vi "Func-엑셀 데이터를 그래프로 출력.vi"() -> ()   [LabVIEW 2015] (continued)
645.21\n645.23\n645.24\n645.26\n645.28\n645.29\n645.31\n645.33\n645.34\n645.36\n645.38\n645.39\n645.41\n645.43\n645.44\n645.46\n645.48\n645.49\n645.51\n645.53\n645.54\n645.56\n645.58\n645.59\n645.61\n645.63\n645.64\n645.66\n645.68\n645.69\n645.71\n645.73\n645.74\n645.76\n645.78\n645.79\n645.81\n645.83\n645.84\n645.86\n645.88\n645.89\n645.91\n645.93\n645.94\n645.96\n645.98\n645.99\n646.01\n646.03\n646.04\n646.06\n646.08\n646.09\n646.11\n646.13\n646.14\n646.16\n646.18\n646.19\n646.21\n646.23\n646.24\n646.26\n646.28\n646.29\n646.31\n646.33\n646.34\n646.36\n646.38\n646.39\n646.41\n646.43\n646.44\n646.46\n646.48\n646.49\n646.51\n646.53\n646.54\n646.56\n646.58\n646.59\n646.61\n646.63\n646.64\n646.66\n646.68\n646.69\n646.71\n646.73\n646.74\n646.76\n646.78\n646.8\n646.81\n646.83\n646.84\n646.86\n646.88\n646.89\n646.91\n646.93\n646.94\n646.96\n646.98\n646.99\n647.01\n647.03\n647.04\n647.06\n647.08\n647.09\n647.11\n647.13\n647.15\n647.16\n647.18\n647.19\n647.21\n647.23\n647.25\n647.26\n647.28\n647.29\n647.31\n647.33\n647.34\n647.36\n647.38\n647.4\n647.41\n647.43\n647.44\n647.46\n647.48\n647.49\n647.51\n647.53\n647.54\n647.56\n647.58\n647.59\n647.61\n647.63\n647.64\n647.66\n647.68\n647.69\n647.71\n647.73\n647.74\n647.76\n647.78\n647.79\n647.81\n647.83\n647.84\n647.86\n647.88\n647.89\n647.91\n647.93\n647.94\n647.96\n647.98\n647.99\n648.01\n648.03\n648.04\n648.06\n648.08\n648.09\n648.11\n648.13\n648.14\n648.16\n648.18\n648.19\n648.21\n648.23\n648.24\n648.26\n648.28\n648.29\n648.31\n648.33\n648.35\n648.36\n648.38\n648.39\n648.41\n648.43\n648.44\n648.46\n648.48\n648.49\n648.51\n648.53\n648.54\n648.56\n648.58\n648.59\n648.61\n648.63\n648.64\n648.66\n648.68\n648.69\n648.71\n648.73\n648.75\n648.76\n648.78\n648.79\n648.81\n648.83\n648.84\n648.86\n648.88\n648.89\n648.91\n648.93\n648.94\n648.96\n648.98\n648.99\n649.01\n649.03\n649.04\n649.06\n649.08\n649.09\n649.11\n649.13\n649.14\n649.16\n649.18\n649.19\n649.21\n649.23\n649.24\n649.26\n649.28\n649.29\n649.31\n649.33\n649.34\n649.36\n649.38\n649.39\n649.41\n649.43\n649.44\n649.46\n649.48\n649.49\n649.51\n649.53\n649.55\n649.56\n649.58\n649.59\n649.61\n649.63\n649.64\n649.66\n649.68\n649.69\n649.71\n649.73\n649.74\n649.76\n649.78\n649.79\n649.81\n649.83\n649.84\n649.86\n649.88\n649.9\n649.91\n649.93\n649.94\n649.96\n649.98\n649.99\n650.01\n650.03\n650.04\n650.06\n650.08\n650.09\n650.11\n650.13\n650.15\n650.16\n650.18\n650.19\n650.21\n650.23\n650.25\n650.26\n650.28\n650.29\n650.31\n650.33\n650.35\n650.36\n650.38\n650.39\n650.41\n650.43\n650.44\n650.46\n650.48\n650.5\n650.51\n650.53\n650.54\n650.56\n650.58\n650.6\n650.61\n650.63\n650.64\n650.66\n650.68\n650.69\n650.71\n650.73\n650.74\n650.76\n650.78\n650.79\n650.81\n650.83\n650.85\n650.86\n650.88\n650.89\n650.91\n650.93\n650.94\n650.96\n650.98\n650.99\n651.01\n651.03\n651.05\n651.06\n651.08\n651.09\n651.11\n651.13\n651.14\n651.16\n651.18\n651.19\n651.21\n651.23\n651.24\n651.26\n651.28\n651.29\n651.31\n651.33\n651.34\n651.36\n651.38\n651.39\n651.41\n651.43\n651.44\n651.46\n651.48\n651.49\n651.51\n651.53\n651.54\n651.56\n651.58\n651.59\n651.61\n651.63\n651.64\n651.66\n651.68\n651.69\n651.71\n651.73\n651.74\n651.76\n651.78\n651.79\n651.81\n651.83\n651.84\n651.86\n651.88\n651.89\n651.91\n651.93\n651.94\n651.96\n651.98\n651.99\n652.01\n652.03\n652.04\n652.06\n652.08\n652.09\n652.11\n652.13\n652.14\n652.16\n652.18\n652.19\n652.21\n652.23\n652.24\n652.26\n652.28\n652.29\n652.31\n652.33\n652.34\n652.36\n652.38\n652.39\n652.41\n652.43\n652.44\n652.46\n652.48\n652.49\n652.51\n652.53\n652.54\n652.56\n652.58\n652.59\n652.61\n652.63\n652.64\n652.66\n652.68\n652.69\n652.71\n652.73\n652.74\n652.76\n652.78\n652.79\n652.81\n652.83\n652.84\n652.86\n652.88\n652.89\n652.91\n652.93\n652.94\n652.96\n652.98\n653\n653.01\n653.03\n653.04\n653.06\n653.08\n653.09\n653.11\n653.13\n653.14\n653.16\n653.18\n653.19\n653.21\n653.23\n653.24\n653.26\n653.28\n653.29\n653.31\n653.33\n653.35\n653.36\n653.38\n653.39\n653.41\n653.43\n653.44\n653.46\n653.48\n653.49\n653.51\n653.53\n653.54\n653.56\n653.58\n653.6\n653.61\n653.63\n653.64\n653.66\n653.68\n653.7\n653.71\n653.73\n653.74\n653.76\n653.78\n653.79\n653.81\n653.83\n653.84\n653.86\n653.88\n653.89\n653.91\n653.93\n653.94\n653.96\n653.98\n653.99\n654.01\n654.03\n654.04\n654.06\n654.08\n654.09\n654.11\n654.13\n654.15\n654.16\n654.18\n654.19\n654.21\n654.23\n654.24\n654.26\n654.28\n654.3\n654.31\n654.33\n654.34\n654.36\n654.38\n654.39\n654.41\n654.43\n654.44\n654.46\n654.48\n654.49\n654.51\n654.53\n654.54\n654.56\n654.58\n654.59\n654.61\n654.63\n654.64\n654.66\n654.68\n654.69\n654.71\n654.73\n654.74\n654.76\n654.78\n654.79\n654.81\n654.83\n654.84\n654.86\n654.88\n654.89\n654.91\n654.93\n654.94\n654.96\n654.98\n654.99\n655.01\n655.03\n655.04\n655.06\n655.08\n655.09\n655.11\n655.13\n655.14\n655.16\n655.18\n655.19\n655.21\n655.23\n655.24\n655.26\n655.28\n655.29\n655.31\n655.33\n655.34\n655.36\n655.38\n655.39\n655.41\n655.43\n655.44\n655.46\n655.48\n655.49\n655.51\n655.53\n655.54\n655.56\n655.58\n655.59\n655.61\n655.63\n655.65\n655.66\n655.68\n655.69\n655.71\n655.73\n655.74\n655.76\n655.78\n655.79\n655.81\n655.83\n655.84\n655.86\n655.88\n655.89\n655.91\n655.93\n655.94\n655.96\n655.98\n655.99\n656.01\n656.03\n656.04\n656.06\n656.08\n656.1\n656.11\n656.13\n656.14\n656.16\n656.18\n656.19\n656.21\n656.23\n656.25\n656.26\n656.28\n656.29\n656.31\n656.33\n656.35\n656.36\n656.38\n656.39\n656.41\n656.43\n656.45\n656.46\n656.48\n656.49\n656.51\n656.53\n656.54\n656.56\n656.58\n656.59\n656.61\n656.63\n656.64\n656.66\n656.68\n656.7\n656.71\n656.73\n656.74\n656.76\n656.78\n656.8\n656.81\n656.83\n656.84\n656.86\n656.88\n656.89\n656.91\n656.93\n656.94\n656.96\n656.98\n656.99\n657.01\n657.03\n657.05\n657.06\n657.08\n657.09\n657.11\n657.13\n657.14\n657.16\n657.18\n657.19\n657.21\n657.23\n657.24\n657.26\n657.28\n657.29\n657.31\n657.33\n657.34\n657.36\n657.38\n657.39\n657.41\n657.43\n657.44\n657.46\n657.48\n657.49\n657.51\n657.53\n657.54\n657.56\n657.58\n657.6\n657.61\n657.63\n657.64\n657.66\n657.68\n657.69\n657.71\n657.73\n657.74\n657.76\n657.78\n657.79\n657.81\n657.83\n657.84\n657.86\n657.88\n657.89\n657.91\n657.93\n657.94\n657.96\n657.98\n657.99\n658.01\n658.03\n658.04\n658.06\n658.08\n658.09\n658.11\n658.13\n658.14\n658.16\n658.18\n658.19\n658.21\n658.23\n658.24\n658.26\n658.28\n658.29\n658.31\n658.33\n658.34\n658.36\n658.38\n658.39\n658.41\n658.43\n658.44\n658.46\n658.48\n658.49\n658.51\n658.53\n658.54\n658.56\n658.58\n658.59\n658.61\n658.63\n658.64\n658.66\n658.68\n658.69\n658.71\n658.73\n658.74\n658.76\n658.78\n658.79\n658.81\n658.83\n658.84\n658.86\n658.88\n658.89\n658.91\n658.93\n658.94\n658.96\n658.98\n658.99\n659.01\n659.03\n659.04\n659.06\n659.08\n659.09\n659.11\n659.13\n659.14\n659.16\n659.18\n659.2\n659.21\n659.23\n659.24\n659.26\n659.28\n659.29\n659.31\n659.33\n659.34\n659.36\n659.38\n659.39\n659.41\n659.43\n659.45\n659.46\n659.48\n659.49\n659.51\n659.53\n659.54\n659.56\n659.58\n659.59\n659.61\n659.63\n659.64\n659.66\n659.68\n659.69\n659.71\n659.73\n659.74\n659.76\n659.78\n659.8\n659.81\n659.83\n659.84\n659.86\n659.88\n659.9\n659.91\n659.93\n659.94\n659.96\n659.98\n659.99\n660.01\n660.03\n660.04\n660.06\n660.08\n660.09\n660.11\n660.13\n660.14\n660.16\n660.18\n660.19\n660.21\n660.23\n660.24\n660.26\n660.28\n660.29\n660.31\n660.33\n660.34\n660.36\n660.38\n660.39\n660.41\n660.43\n660.44\n660.46\n660.48\n660.5\n660.51\n660.53\n660.54\n660.56\n660.58\n660.59\n660.61\n660.63\n660.65\n660.66\n660.68\n660.69\n660.71\n660.73\n660.74\n660.76\n660.78\n660.79\n660.81\n660.83\n660.84\n660.86\n660.88\n660.89\n660.91\n660.93\n660.94\n660.96\n660.98\n660.99\n661.01\n661.03\n661.04\n661.06\n661.08\n661.09\n661.11\n661.13\n661.14\n661.16\n661.18\n661.19\n661.21\n661.23\n661.24\n661.26\n661.28\n661.29\n661.31\n661.33\n661.34\n661.36\n661.38\n661.39\n661.41\n661.43\n661.44\n661.46\n661.48\n661.49\n661.51\n661.53\n661.54\n661.56\n661.58\n661.59\n661.61\n661.63\n661.64\n661.66\n661.68\n661.69\n661.71\n661.73\n661.75\n661.76\n661.78\n661.79\n661.81\n661.83\n661.84\n661.86\n661.88\n661.89\n661.91\n661.93\n661.94\n661.96\n661.98\n661.99\n662.01\n662.03\n662.04\n662.06\n662.08\n662.09\n662.11\n662.13\n662.14\n662.16\n662.18\n662.2\n662.21\n662.23\n662.24\n662.26\n662.28\n662.29\n662.31\n662.33\n662.35\n662.36\n662.38\n662.39\n662.41\n662.43\n662.45\n662.46\n662.48\n662.49\n662.51\n662.53\n662.55\n662.56\n662.58\n662.59\n662.61\n662.63\n662.64\n662.66\n662.68\n662.69\n662.71\n662.73\n662.74\n662.76\n662.78\n662.8\n662.81\n662.83\n662.84\n662.86\n662.88\n662.9\n662.91\n662.93\n662.95\n662.96\n662.98\n662.99\n663.01\n663.03\n663.04\n663.06\n663.08\n663.09\n663.11\n663.13\n663.15\n663.16\n663.18\n663.19\n663.21\n663.23\n663.24\n663.26\n663.28\n663.29\n663.31\n663.33\n663.34\n663.36\n663.38\n663.4\n663.41\n663.43\n663.44\n663.46\n663.48\n663.49\n663.51\n663.53\n663.54\n663.56\n663.58\n663.59\n663.61\n663.63\n663.64\n663.66\n663.68\n663.7\n663.71\n663.73\n663.74\n663.76\n663.78\n663.79\n663.81\n663.83\n663.84\n663.86\n663.88\n663.89\n663.91\n663.93\n663.94\n663.96\n663.98\n664\n664.01\n664.03\n664.04\n664.06\n664.08\n664.09\n664.11\n664.13\n664.14\n664.16\n664.18\n664.19\n664.21\n664.23\n664.24\n664.26\n664.28\n664.29\n664.31\n664.33\n664.34\n664.36\n664.38\n664.39\n664.41\n664.43\n664.44\n664.46\n664.48\n664.49\n664.51\n664.53\n664.54\n664.56\n664.58\n664.59\n664.61\n664.63\n664.64\n664.66\n664.68\n664.69\n664.71\n664.73\n664.74\n664.76\n664.78\n664.79\n664.81\n664.83\n664.84\n664.86\n664.88\n664.89\n664.91\n664.93\n664.94\n664.96\n664.98\n664.99\n665.01\n665.03\n665.04\n665.06\n665.08\n665.09\n665.11\n665.13\n665.14\n665.16\n665.18\n665.2\n665.21\n665.23\n665.24\n665.26\n665.28\n665.29\n665.31\n665.33\n665.34\n665.36\n665.38\n665.39\n665.41\n665.43\n665.44\n665.46\n665.48\n665.49\n665.51\n665.53\n665.55\n665.56\n665.58\n665.59\n665.61\n665.63\n665.65\n665.66\n665.68\n665.69\n665.71\n665.73\n665.74\n665.76\n665.78\n665.8\n665.81\n665.83\n665.84\n665.86\n665.88\n665.9\n665.91\n665.93\n665.94\n665.96\n665.98\n666\n666.01\n666.03\n666.04\n666.06\n666.08\n666.09\n666.11\n666.13\n666.15\n666.16\n666.18\n666.19\n666.21\n666.23\n666.25\n666.26\n666.28\n666.29\n666.31\n666.33\n666.35\n666.36\n666.38\n666.39\n666.41\n666.43\n666.44\n666.46\n666.48\n666.49\n666.51\n666.53\n666.54\n666.56\n666.58\n666.59\n666.61\n666.63\n666.64\n666.66\n666.68\n666.69\n666.71\n666.73\n666.74\n666.76\n666.78\n666.79\n666.81\n666.83\n666.84\n666.86\n666.88\n666.89\n666.91\n666.93\n666.94\n666.96\n666.98\n666.99\n667.01\n667.03\n667.04\n667.06\n667.08\n667.09\n667.11\n667.13\n667.14\n667.16\n667.18\n667.19\n667.21\n667.23\n667.24\n667.26\n667.28\n667.29\n667.31\n667.33\n667.34\n667.36\n667.38\n667.39\n667.41\n667.43\n667.44\n667.46\n667.48\n667.49\n667.51\n667.53\n667.54\n667.56\n667.58\n667.59\n667.61\n667.63\n667.64\n667.66\n667.68\n667.69\n667.71\n667.73\n667.74\n667.76\n667.78\n667.79\n667.81\n667.83\n667.84\n667.86\n667.88\n667.89\n667.91\n667.93\n667.94\n667.96\n667.98\n667.99\n668.01\n668.03\n668.04\n668.06\n668.08\n668.09\n668.11\n668.13\n668.14\n668.16\n668.18\n668.19\n668.21\n668.23\n668.24\n668.26\n668.28\n668.29\n668.31\n668.33\n668.34\n668.36\n668.38\n668.39\n668.41\n668.43\n668.44\n668.46\n668.48\n668.49\n668.51\n668.53\n668.54\n668.56\n668.58\n668.59\n668.61\n668.63\n668.65\n668.66\n668.68\n668.69\n668.71\n668.73\n668.75\n668.76\n668.78\n668.79\n668.81\n668.83\n668.84\n668.86\n668.88\n668.89\n668.91\n668.93\n668.94\n668.96\n668.98\n669\n669.01\n669.03\n669.04\n669.06\n669.08\n669.1\n669.11\n669.13\n669.14\n669.16\n669.18\n669.19\n669.21\n669.23\n669.24\n669.26\n669.28\n669.29\n669.31\n669.33\n669.34\n669.36\n669.38\n669.39\n669.41\n669.43\n669.44\n669.46\n669.48\n669.49\n669.51\n669.53\n669.54\n669.56\n669.58\n669.59\n669.61\n669.63\n669.64\n669.66\n669.68\n669.69\n669.71\n669.73\n669.74\n669.76\n669.78\n669.8\n669.81\n669.83\n669.84\n669.86\n669.88\n669.89\n669.91\n669.93\n669.94\n669.96\n669.98\n669.99\n670.01\n670.03\n670.04\n670.06\n670.08\n670.09\n670.11\n670.13\n670.14\n670.16\n670.18\n670.2\n670.21\n670.23\n670.24\n670.26\n670.28\n670.29\n670.31\n670.33\n670.34\n670.36\n670.38\n670.39\n670.41\n670.43\n670.44\n670.46\n670.48\n670.49\n670.51\n670.53\n670.54\n670.56\n670.58\n670.59\n670.61\n670.63\n670.64\n670.66\n670.68\n670.7\n670.71\n670.73\n670.74\n670.76\n670.78\n670.79\n670.81\n670.83\n670.84\n670.86\n670.88\n670.89\n670.91\n670.93\n670.94\n670.96\n670.98\n670.99\n671.01\n671.03\n671.04\n671.06\n671.08\n671.09\n671.11\n671.13\n671.14\n671.16\n671.18\n671.19\n671.21\n671.23\n671.24\n671.26\n671.28\n671.3\n671.31\n671.33\n671.34\n671.36\n671.38\n671.39\n671.41\n671.43\n671.44\n671.46\n671.48\n671.49\n671.51\n671.53\n671.54\n671.56\n671.58\n671.59\n671.61\n671.63\n671.64\n671.66\n671.68\n671.69\n671.71\n671.73\n671.75\n671.76\n671.78\n671.79\n671.81\n671.83\n671.85\n671.86\n671.88\n671.9\n671.91\n671.93\n671.94\n671.96\n671.98\n671.99\n672.01\n672.03\n672.04\n672.06\n672.08\n672.1\n672.11\n672.13\n672.14\n672.16\n672.18\n672.2\n672.21\n672.23\n672.24\n672.26\n672.28\n672.29\n672.31\n672.33\n672.35\n672.36\n672.38\n672.39\n672.41\n672.43\n672.44\n672.46\n672.48\n672.49\n672.51\n672.53\n672.54\n672.56\n672.58\n672.59\n672.61\n672.63\n672.64\n672.66\n672.68\n672.69\n672.71\n672.73\n672.74\n672.76\n672.78\n672.79\n672.81\n672.83\n672.84\n672.86\n672.88\n672.89\n672.91\n672.93\n672.95\n672.96\n672.98\n672.99\n673.01\n673.03\n673.04\n673.06\n673.08\n673.09\n673.11\n673.13\n673.14\n673.16\n673.18\n673.19\n673.21\n673.23\n673.24\n673.26\n673.28\n673.29\n673.31\n673.33\n673.34\n673.36\n673.38\n673.39\n673.41\n673.43\n673.44\n673.46\n673.48\n673.49\n673.51\n673.53\n673.54\n673.56\n673.58\n673.59\n673.61\n673.63\n673.64\n673.66\n673.68\n673.69\n673.71\n673.73\n673.74\n673.76\n673.78\n673.79\n673.81\n673.83\n673.84\n673.86\n673.88\n673.89\n673.91\n673.93\n673.94\n673.96\n673.98\n673.99\n674.01\n674.03\n674.04\n674.06\n674.08\n674.09\n674.11\n674.13\n674.14\n674.16\n674.18\n674.19\n674.21\n674.23\n674.24\n674.26\n674.28\n674.29\n674.31\n674.33\n674.34\n674.36\n674.38\n674.39\n674.41\n674.43\n674.44\n674.46\n674.48\n674.5\n674.51\n674.53\n674.54\n674.56\n674.58\n674.59\n674.61\n674.63\n674.64\n674.66\n674.68\n674.69\n674.71\n674.73\n674.75\n674.76\n674.78\n674.79\n674.81\n674.83\n674.85\n674.86\n674.88\n674.89\n674.91\n674.93\n674.95\n674.96\n674.98\n674.99\n675.01\n675.03\n675.04\n675.06\n675.08\n675.09\n675.11\n675.13\n675.14\n675.16\n675.18\n675.2\n675.21\n675.23\n675.24\n675.26\n675.28\n675.3\n675.31\n675.33\n675.35\n675.36\n675.38\n675.39\n675.41\n675.43\n675.45\n675.46\n675.48\n675.49\n675.51\n675.53\n675.54\n675.56\n675.58\n675.59\n675.61\n675.63\n675.64\n675.66\n675.68\n675.69\n675.71\n675.73\n675.74\n675.76\n675.78\n675.79\n675.81\n675.83\n675.84\n675.86\n675.88\n675.89\n675.91\n675.93\n675.94\n675.96\n675.98\n675.99\n676.01\n676.03\n676.04\n676.06\n676.08\n676.09\n676.11\n676.13\n676.14\n676.16\n676.18\n676.19\n676.21\n676.23\n676.24\n676.26\n676.28\n676.29\n676.31\n676.33\n676.34\n676.36\n676.38\n676.39\n676.41\n676.43\n676.44\n676.46\n676.48\n676.49\n676.51\n676.53\n676.54\n676.56\n676.58\n676.59\n676.61\n676.63\n676.64\n676.66\n676.68\n676.69\n676.71\n676.73\n676.74\n676.76\n676.78\n676.79\n676.81\n676.83\n676.84\n676.86\n676.88\n676.89\n676.91\n676.93\n676.94\n676.96\n676.98\n676.99\n677.01\n677.03\n677.04\n677.06\n677.08\n677.09\n677.11\n677.13\n677.14\n677.16\n677.18\n677.19\n677.21\n677.23\n677.25\n677.26\n677.28\n677.29\n677.31\n677.33\n677.34\n677.36\n677.38\n677.39\n677.41\n677.43\n677.44\n677.46\n677.48\n677.49\n677.51\n677.53\n677.54\n677.56\n677.58\n677.6\n677.61\n677.63\n677.64\n677.66\n677.68\n677.69\n677.71\n677.73\n677.74\n677.76\n677.78\n677.79\n677.81\n677.83\n677.84\n677.86\n677.88\n677.89\n677.91\n677.93\n677.95\n677.96\n677.98\n677.99\n678.01\n678.03\n678.04\n678.06\n678.08\n678.09\n678.11\n678.13\n678.14\n678.16\n678.18\n678.19\n678.21\n678.23\n678.24\n678.26\n678.28\n678.3\n678.31\n678.33\n678.34\n678.36\n678.38\n678.39\n678.41\n678.43\n678.44\n678.46\n678.48\n678.49\n678.51\n678.53\n678.54\n678.56\n678.58\n678.59\n678.61\n678.63\n678.65\n678.66\n678.68\n678.69\n678.71\n678.73\n678.74\n678.76\n678.78\n678.79\n678.81\n678.83\n678.84\n678.86\n678.88\n678.9\n678.91\n678.93\n678.94\n678.96\n678.98\n679\n679.01\n679.03\n679.04\n679.06\n679.08\n679.09\n679.11\n679.13\n679.14\n679.16\n679.18\n679.19\n679.21\n679.23\n679.24\n679.26\n696.27\n696.44\n696.61\n696.77\n696.94\n697.11\n697.27\n697.44\n697.61\n697.77\n697.94\n698.11\n698.27\n698.44\n698.61\n698.77\n698.94\n699.11\n699.27\n699.44\n699.61\n699.77\n699.94\n700.11\n700.27\n700.44\n700.61\n700.77\n700.94\n701.11\n701.27\n701.44\n701.61\n701.77\n701.94\n702.11\n702.27\n702.44\n702.61\n702.77\n702.94\n703.11\n703.27\n703.44\n703.61\n703.77\n703.94\n704.11\n704.28\n704.45\n704.61\n704.78\n704.95\n705.11\n705.28\n705.45\n705.61\n705.78\n705.95\n706.11\n706.28\n706.45\n706.62\n706.78\n706.95\n707.12\n707.28\n707.45\n707.61\n707.78\n707.95\n708.11\n708.28\n708.45\n708.61\n708.78\n708.95\n709.11\n709.28\n709.45\n709.62\n709.78\n709.95\n710.11\n710.28\n710.45\n710.61\n710.78\n710.95\n711.12\n711.29\n711.46\n711.62\n711.79\n711.96\n712.12\n712.29\n712.46\n712.62\n712.79\n712.96\n713.12\n713.29\n713.46\n713.62\n713.79\n713.96\n714.12\n714.29\n714.46\n714.62\n714.79\n714.96\n715.13\n715.3\n715.47\n715.63\n715.8\n715.96\n716.13\n716.3\n716.46\n716.63\n716.8\n716.96\n717.13\n717.3\n717.46\n717.63\n717.8\n717.96\n718.13\n718.3\n718.47\n718.63\n718.8\n718.96\n719.13\n719.3\n719.46\n719.63\n719.8\n719.96\n720.13\n720.3\n720.46\n720.63\n720.8\n720.96\n721.13\n721.3\n721.46\n721.63\n721.8\n721.96\n722.13\n722.3\n722.46\n722.63\n722.8\n722.96\n723.13\n723.3\n723.46\n723.63\n723.8\n723.96\n724.13\n724.3\n724.46\n724.63\n724.8\n724.96\n725.13\n725.3\n725.46\n725.63\n725.8\n725.96\n726.13\n726.3\n726.46\n726.63\n726.8\n726.96\n727.13\n727.3\n727.47\n727.64\n727.81\n727.97\n728.14\n728.31\n728.47\n728.64\n728.81\n728.97\n729.14\n729.31\n729.47\n729.64\n729.81\n729.97\n730.14\n730.31\n730.47\n730.64\n730.81\n730.97\n731.14\n731.31\n731.47\n731.64\n731.81\n731.97\n732.14\n732.31\n732.47\n732.64\n732.81\n732.97\n733.14\n733.31\n733.48\n733.65\n733.81\n733.98\n734.15\n734.32\n734.48\n734.65\n734.81\n734.98\n735.15\n735.31\n735.48\n735.65\n735.81\n735.98\n736.15\n736.32\n736.48\n736.49\n736.51\n736.53\n736.54\n736.56\n736.58\n736.6\n736.61\n736.63\n736.64\n736.66\n736.68\n736.7\n736.71\n736.73\n736.74\n736.76\n736.78\n736.79\n736.81\n736.83\n736.84\n736.86\n736.88\n736.89\n736.91\n736.93\n736.94\n736.96\n736.98\n736.99\n737.01\n737.03\n737.05\n737.06\n737.08\n737.09\n737.11\n737.13\n737.14\n737.16\n737.18\n737.19\n737.21\n737.23\n737.24\n737.26\n737.28\n737.3\n737.31\n737.33\n737.34\n737.36\n737.38\n737.4\n737.41\n737.43\n737.44\n737.46\n737.48\n737.49\n737.51\n737.53\n737.54\n737.56\n737.58\n737.59\n737.61\n737.63\n737.64\n737.66\n737.68\n737.69\n737.71\n737.73\n737.75\n737.76\n737.78\n737.79\n737.81\n737.83\n737.84\n737.86\n737.88\n737.9\n737.91\n737.93\n737.94\n737.96\n737.98\n737.99\n738.01\n738.03\n738.04\n738.06\n738.08\n738.09\n738.11\n738.13\n738.14\n738.16\n738.18\n738.19\n738.21\n738.23\n738.25\n738.26\n738.28\n738.29\n738.31\n738.33\n738.35\n738.36\n738.38\n738.39\n738.41\n738.43\n738.44\n738.46\n738.48\n738.49\n738.51\n738.53\n738.54\n738.56\n738.58\n738.59\n738.61\n738.63\n738.64\n738.66\n738.68\n738.69\n738.71\n738.73\n738.74\n738.76\n738.78\n738.79\n738.81\n738.83\n738.84\n738.86\n738.88\n738.89\n738.91\n738.93\n738.94\n738.96\n738.98\n738.99\n739.01\n739.03\n739.04\n739.06\n739.08\n739.09\n739.11\n739.13\n739.14\n739.16\n739.18\n739.19\n739.21\n739.23\n739.24\n739.26\n739.28\n739.29\n739.31\n739.33\n739.34\n739.36\n739.38\n739.39\n739.41\n739.43\n739.44\n739.46\n739.48\n739.49\n739.51\n739.53\n739.54\n739.56\n739.58\n739.59\n739.61\n739.63\n739.64\n739.66\n739.68\n739.69\n739.71\n739.73\n739.74\n739.76\n739.78\n739.79\n739.81\n739.83\n739.84\n739.86\n739.88\n739.89\n739.91\n739.93\n739.94\n739.96\n739.98\n739.99\n740.01\n740.03\n740.05\n740.06\n740.08\n740.09\n740.11\n740.13\n740.14\n740.16\n740.18\n740.19\n740.21
